vi "Timestamped CSV.vi"(11 "Comma-separated Text":string) -> ()   [LabVIEW 2011]
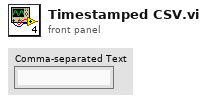
[diagram p1: front panel]
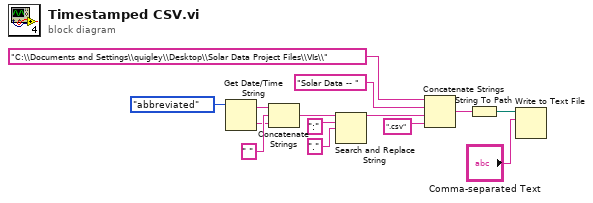
[diagram p0: block diagram]
diagram:
  n1 = Get Date/Time String(date format (0)=enum16{"short", "long", "abbreviated"}."abbreviated") -> (date string=w6:string, time string=w7:string)  [unwired: 2 in]
  n2 = Concatenate Strings(w6, " " ("string"), w7) -> (w10:string)
  n3 = Search and Replace String(input string=w10, search string=":", replace string="." ("replace string (\"\")")) -> (result string=w9:string)  [unwired: 5 in, 3 out]
  n4 = Concatenate Strings("C:\\Documents and Settings\\quigley\\Desktop\\Solar Data Project Files\\VIs\\", "Solar Data -- ", w9, ".csv" ("string")) -> (w14:string)
  n5 = String To Path(string=w14) -> (path=w2:path)
  n6 = Write to Text File(file (use dialog)=w2, text="Comma-separated Text") -> ()  [unwired: 2 in, 3 out]
